vi "FTW-JSON-Construct-FromBuffer.vi"(5 "JSON String (UTF-8)":string, 11 "error in":errorcluster) -> (4 "JSON Object":refnum<class "FTW-JSON.lvclass">, 15 "error out":errorcluster)   [LabVIEW 2013, in "FTW-JSON.lvclass"]
uses:
  FTW-JSON.lvclass
  FTW-JSON.lvclass/FTW-JSON.ctl
panel:
  # "Inputs"
  # "Outputs"
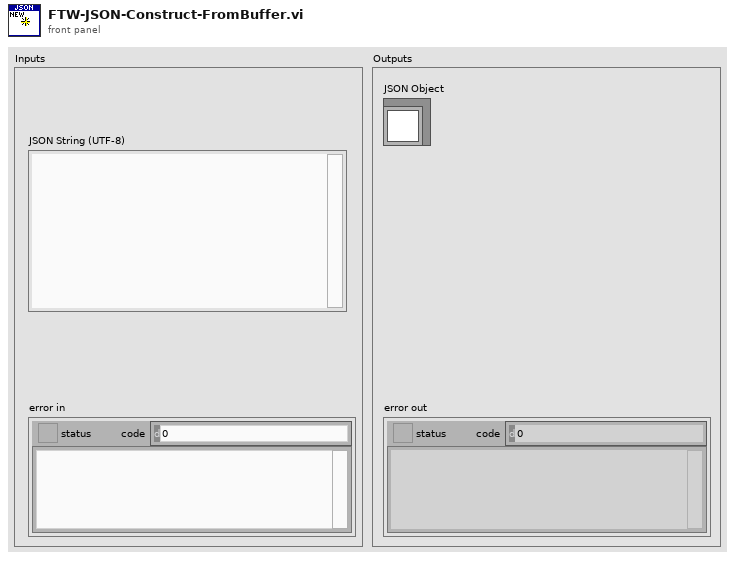
[diagram p1: front panel]
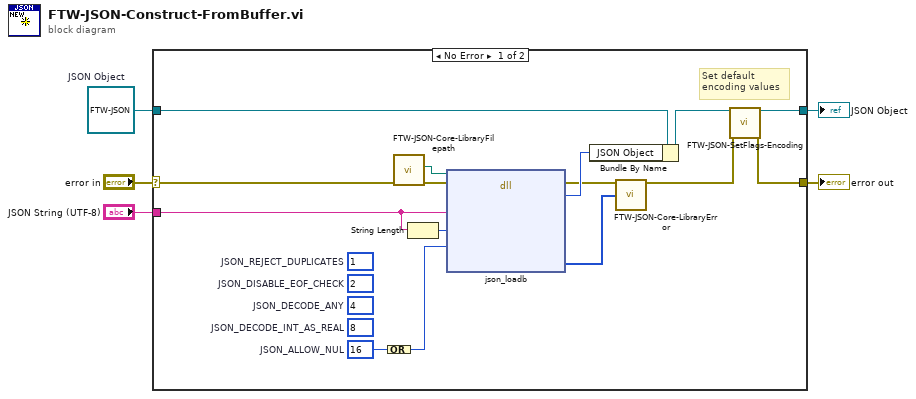
[diagram p0: block diagram]
diagram:
  w4 = refnum<class "FTW-JSON.lvclass"> refnum  # JSON Object
  n1 = case shown="No Error" "error in" {
    selector: "error in" -> [w19 w22]
    tunnel: [w6 w22] -> w5
    tunnel: [w8 w21] -> w3
    tunnel: w4 -> [w20 w21]
    tunnel: "JSON String (UTF-8)" -> [w13 _]
    frame No Error {
      w10 = u64 16  # JSON_ALLOW_NUL
      (unwired) u64 8  # JSON_DECODE_INT_AS_REAL
      (unwired) u64 4  # JSON_DECODE_ANY
      (unwired) u64 2  # JSON_DISABLE_EOF_CHECK
      (unwired) u64 1  # JSON_REJECT_DUPLICATES
      # "Set default\nencoding values"
      n2 = Compound Arithmetic op=OR(w10) -> (w11:u64)
      n3 = call "FTW-JSON-Core-LibraryFilepath.vi"("error in"=w19) -> ("error out"=w18:errorcluster, "JSON Library Filepath"=w17:path)  [unwired: 9 in]
      n4 = String Length(string=w13) -> (length=w12:i32)
      n5 = dll-call lib="?" fn="json_loadb"(path in=w17, error in=w18, "JSON Buffer"=w13, "Buffer Size"=w12, "Flags"=w11) -> (error out=w15:errorcluster, "JSON Object Pointer"=w16:i64, "Error Structure"=w14:u8[])  [unwired: 5 in, 1 out]
      n6 = Bundle By Name(cluster=w20, "JSON Object"=w16) -> (w9:refnum<class "FTW-JSON.lvclass">)
      n7 = call "FTW-JSON-Core-LibraryError.vi"("error in"=w15, "Error Structure"=w14) -> ("error out"=w7:errorcluster)  [unwired: 13 in]
      n8 = call "FTW-JSON-SetFlags-Encoding.vi"("JSON Object"=w9, "error in"=w7) -> ("JSON Object out"=w8:refnum<class "FTW-JSON.lvclass">, "error out"=w6:errorcluster)  [unwired: 12 in]
    }
    frame Error {
    }
  }
  "error out" <- w5
  "JSON Object" <- w3
